vi "Configuration Window.vi"(8 "error in (no error)":errorcluster, 11 "Instrument.Lockin":refnum<class "Instrument.Lockin.lvclass">) -> (0 "error out":errorcluster, 3 "Instrument.Lockin out":refnum<class "Instrument.Lockin.lvclass">)   [LabVIEW 2019, in "Instrument.Lockin.lvlib" / "Instrument.Lockin.lvclass"]
uses:
  Instrument.Lockin.lvclass
  <userlib>/LevyLab/Instrument Framework/Instrument Types/Lockin/Instrument.LockinAPI.lvclass
panel:
  in  "Cancel":bool
  in  "OK":bool
  # "confirm or make changes:"
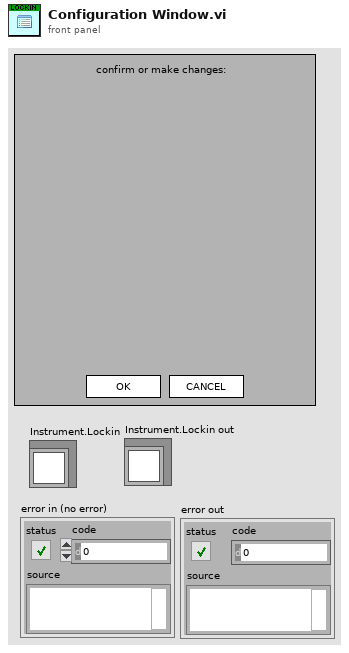
[diagram p1: front panel]
types:
  T1 = enum32{"Invalid", "Standard", "Closed", "Hidden", "Minimized", "Maximized"}
  T2 = enum32{"invalid app kind", "Development System", "Run Time System", "Student Edition", "Embedded LabVIEW", "Evaluation", "Custom"}
  T3 = typedef "Instrument.Lockin.lvlib/Instrument.DAQ.lvclass/Configuration--Cluster.ctl" = cluster{"DAQ":T4, "Channels":T19, "Prefilter":T27, "Offset and Gain":T28, "Amplitude Limit":T31, "DC Limit":T32, "Link Frequencies":T33, "Sweep":T34, "Duty Cycle":T38}
  T4 = typedef "Instrument.Lockin.lvlib/Instrument.DAQ.lvclass/Configuration.DAQ--Cluster.ctl" = cluster{"Sampling":T5, "Simulation mode":T8, "AI":T9, "AO":T14, "Calibration":T16, "Devices":T18[]}
  T5 = typedef "Instrument.Lockin.lvlib/Instrument.DAQ.lvclass/DAQ.Sampling--Cluster.ctl" = cluster{"Sampling":T6, "sample mode":i32, "Fs Mode":T7, "Fs Multiplier":dbl, "Refresh Rate (Hz)":dbl, "Decimation.PreDSP":i32, "Decimation.PostDSP":i32, "Fs.Output":dbl}
  T6 = typedef "Instrument.Lockin.lvlib/Instrument.DAQ.lvclass/DAQ.Sampling.Sampling--Cluster.ctl" = cluster{"Fs":dbl, "#s":i32}
  T7 = typedef "Instrument.Lockin.lvlib/Instrument.DAQ.lvclass/DAQ.Sampling.Fs Mode--enum.ctl" = enum16{"Manual", "Auto Fs", "Max Fs"}
  T8 = typedef "Instrument.Lockin.lvlib/Instrument.DAQ.lvclass/Simulation Mode--enum.ctl" = enum16{"AI = HW simulated", "AI = noise*AO", "AI = waveguide"}
  T9 = typedef "Instrument.Lockin.lvlib/Instrument.DAQ.lvclass/DAQ.Config.AI--Cluster--Array.ctl" = cluster{"Channels":tag, "Coupling":T10, "Range":T11, "terminal configuration":T12, "Type":T13}[]
  T10 = typedef "Instrument.Lockin.lvlib/Instrument.DAQ.lvclass/DAQ.Config.AI.Coupling--enum.ctl" = u16
  T11 = typedef "Instrument.Lockin.lvlib/Instrument.DAQ.lvclass/DAQ.Config.AI.Range--enum.ctl" = enum16{"±0.316", "±1.00", "±3.16", "±10.0", "±31.6", "±42.4", ""}
  T12 = typedef "Instrument.Lockin.lvlib/Instrument.DAQ.lvclass/DAQ.TerminalConfiguration--ring.ctl" = i32
  T13 = typedef "Instrument.Lockin.lvlib/Instrument.DAQ.lvclass/DAQ.Type--enum.ctl" = enum16{"None", "USB-4431", "PXI-446x"}
  T14 = typedef "Instrument.Lockin.lvlib/Instrument.DAQ.lvclass/DAQ.Config.AO--Cluster--Array.ctl" = cluster{"Channels":tag, "Range":T15, "terminal configuration":T12, "Type":T13}[]
  T15 = typedef "Instrument.Lockin.lvlib/Instrument.DAQ.lvclass/DAQ.Config.AO.Range--enum.ctl" = enum16{"±0.1", "±1.0", "±3.5", "±10.0", ""}
  T16 = typedef "Instrument.Lockin.lvlib/Instrument.DAQ.lvclass/DAQ.Calibration--Cluster--Array.ctl" = T17[]
  T17 = typedef "Instrument.Lockin.lvlib/Instrument.DAQ.lvclass/DAQ.Calibration--Cluster.ctl" = cluster{"Active Device":string, "SelfCal.LastDate/Time":dbl, "SelfCal.LastTemp":dbl, "DevTemp":dbl, "calibration due?":bool}
  T18 = typedef "Instrument.Lockin.lvlib/Instrument.DAQ.lvclass/DeviceInfo--Cluster.ctl" = cluster{"DeviceName":string, "DevIsSimulated":bool, "DeviceSerialNumber":string, "ProductType":string, "ProductCategory":i32, "ProductNumber":u32, "ChassisNumber":u32, "SlotNumber":u32, "ChassisName":string, "ChassisSerialNumber":string, "DevTemp":dbl, "SelfCal.LastDate/Time":string, "SelfCal.LastTemp":dbl, "calibration due?":bool}
  T19 = typedef "Instrument.Lockin.lvlib/Instrument.DAQ.lvclass/Configuration.Channels--Cluster.ctl" = cluster{"Cfg_AO":T20, "Cfg_AI":T23, "Cfg_REF":T25}
  T20 = typedef "Instrument.Lockin.lvlib/Instrument.DAQ.lvclass/AO.Channel--Cluster--Array.ctl" = T21[]
  T21 = typedef "Instrument.Lockin.lvlib/Instrument.DAQ.lvclass/AO.Channel--Cluster.ctl" = cluster{"Enable?":bool, "Channel":i32, "Amplitude":dbl, "Offset":dbl, "Frequency":dbl, "Phase":dbl, "Function":T22, "Sweeping?":bool, "Limit AC":bool, "Limit DC?":bool, "Duty Cycle":bool}
  T22 = typedef "Instrument.Lockin.lvlib/Instrument.DAQ.lvclass/AO.Channel.Function--Enum.ctl" = enum16{"sine", "square", "triangle", "saw"}
  T23 = typedef "Instrument.Lockin.lvlib/Instrument.DAQ.lvclass/AI.Channel--Cluster--Array.ctl" = T24[]
  T24 = typedef "Instrument.Lockin.lvlib/Instrument.DAQ.lvclass/AI.Channel--Cluster.ctl" = cluster{"Enable?":bool, "Channel":i32, "References":u16[], "reference index":i32}
  T25 = typedef "Instrument.Lockin.lvlib/Instrument.DAQ.lvclass/REF.Channel--Cluster--Array.ctl" = T26[]
  T26 = typedef "Instrument.Lockin.lvlib/Instrument.DAQ.lvclass/REF.Channel--Cluster.ctl" = cluster{"Enable?":bool, "Channel":i32, "Frequency":dbl, "Phase":dbl, "TC":dbl, "Roll-Off":i32}
  T27 = typedef "Instrument.Lockin.lvlib/Instrument.DAQ.lvclass/Configuration.Prefilter--Cluster.ctl" = cluster{"60 Hz":bool, "Low Pass":bool, "Low Pass Cutoff (Hz)":dbl}
  T28 = typedef "Instrument.Lockin.lvlib/Instrument.DAQ.lvclass/Channel.GainsAndOffsets--Cluster.ctl" = cluster{"Offset_AI":T29, "Gain_AI":T29, "Gain_AO":T29}
  T29 = typedef "Instrument.Lockin.lvlib/Instrument.DAQ.lvclass/Channel.Gain--Cluster--Array.ctl" = T30[]
  T30 = typedef "Instrument.Lockin.lvlib/Instrument.DAQ.lvclass/Channel.Gain--Cluster.ctl" = cluster{"Channel":string, "Gain":dbl}
  T31 = typedef "Instrument.Lockin.lvlib/Instrument.DAQ.lvclass/Configuration.AmplitudeLimit--Cluster.ctl" = cluster{"Limit?":bool, "Limit (V)":dbl}
  T32 = typedef "Instrument.Lockin.lvlib/Instrument.DAQ.lvclass/Configuration.DCLimit--Cluster.ctl" = cluster{"Limit?":bool, "Limit (V)":dbl}
  T33 = typedef "Instrument.Lockin.lvlib/Instrument.DAQ.lvclass/Configuration.LinkFrequencies--Cluster.ctl" = cluster{"Link?":bool, "Frequency (Hz)":dbl}
  T34 = typedef "Instrument.Lockin.lvlib/Instrument.DAQ.lvclass/Sweep.Configuration--Cluster.ctl" = cluster{"Sweep Time (s)":dbl, "Initial Wait (s)":dbl, "Return to Start":bool, "Channels":T35}
  T35 = typedef "Instrument.Lockin.lvlib/Instrument.DAQ.lvclass/Sweep.Channel--Cluster--Array.ctl" = T36[]
  T36 = typedef "Instrument.Lockin.lvlib/Instrument.DAQ.lvclass/Sweep.Channel--Cluster.ctl" = cluster{"Enable?":bool, "Channel":u16, "Start":dbl, "End":dbl, "Pattern":T37, "Table":dbl[]}
  T37 = typedef "Instrument.Lockin.lvlib/Instrument.DAQ.lvclass/Sweep.Pattern--Enum.ctl" = enum16{"Ramp /", "Ramp /\\", "Smooth Ramp _/", "Smooth Ramp _/\\_", "Table"}
  T38 = typedef "Instrument.Lockin.lvlib/Instrument.DAQ.lvclass/Configuration.DutyCycle--Cluster.ctl" = cluster{"Option?":bool, "Duty Cycle (%)":dbl}
  T39 = cluster{"Core":cluster{"Current VI Reference":refnum<vi>, "Close Panel on Exit?":bool}, "Configuration":T3}
  T40 = cluster{"Current VI Reference":refnum<vi>, "Close Panel on Exit?":bool}
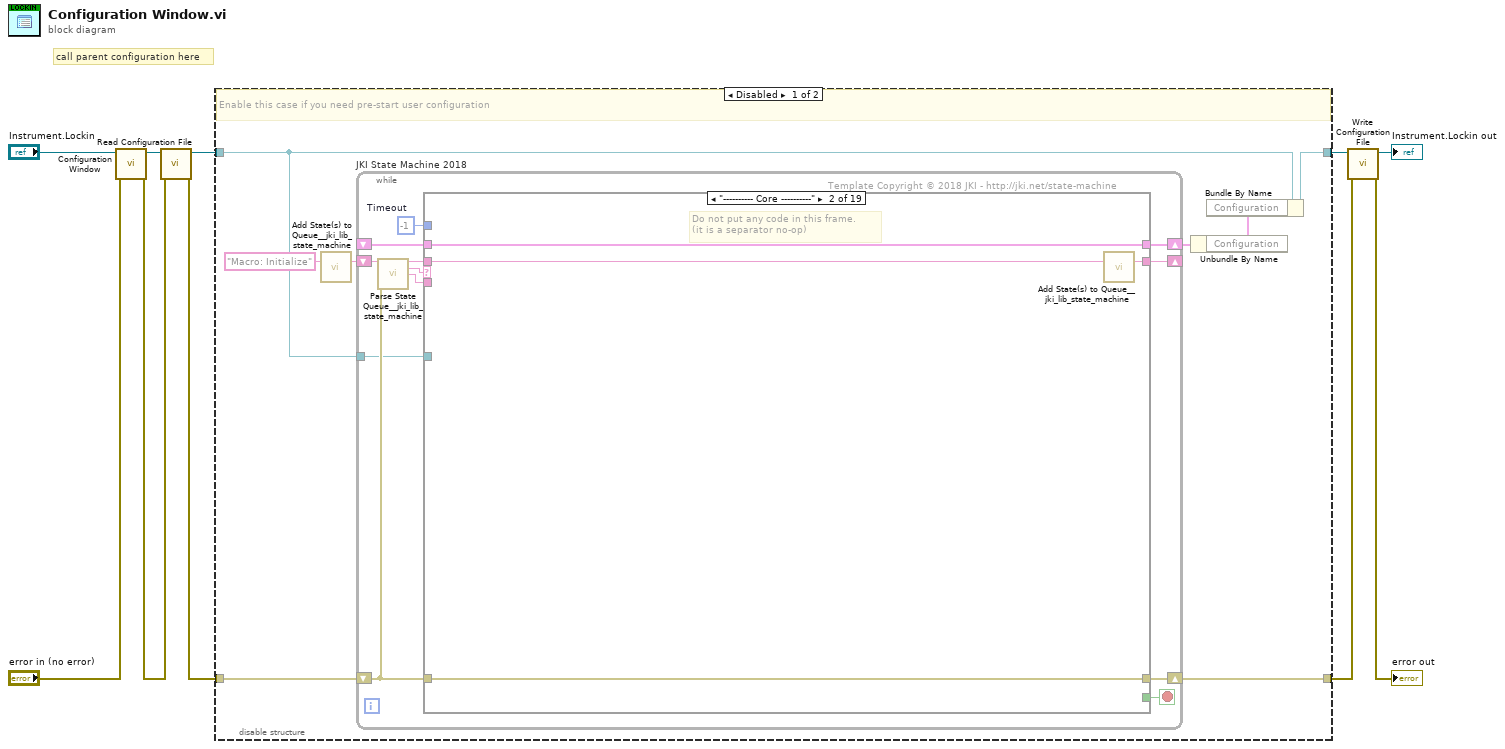
[diagram p0: block diagram]
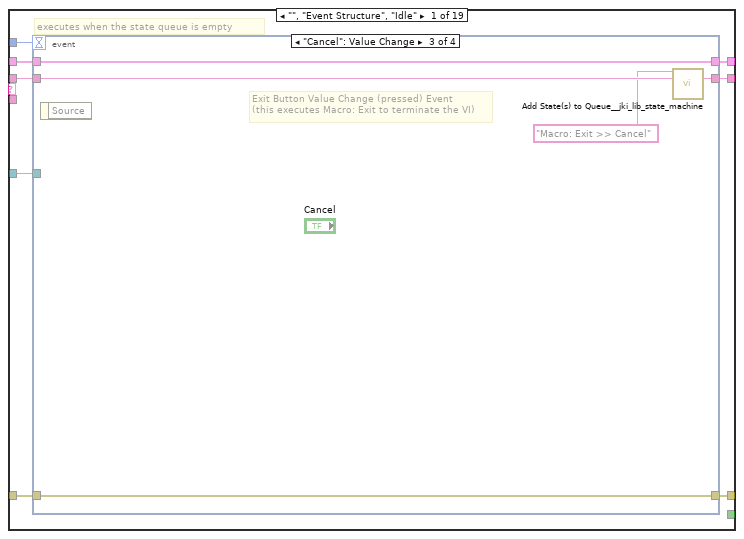
[diagram p2: hidden frame]
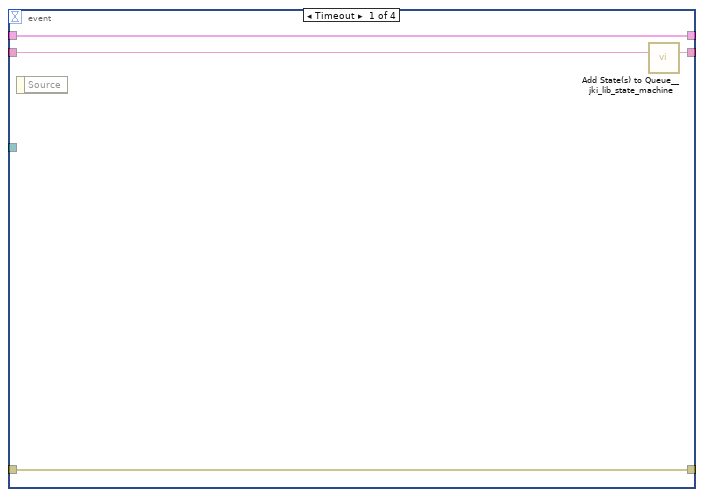
[diagram p3: hidden frame]
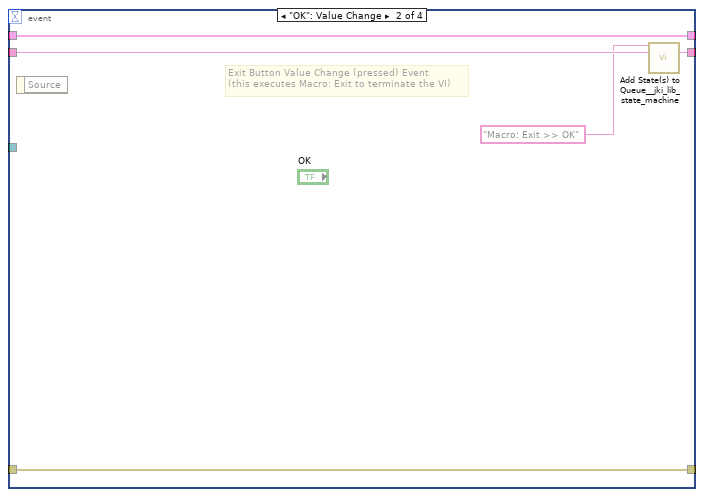
[diagram p4: hidden frame]
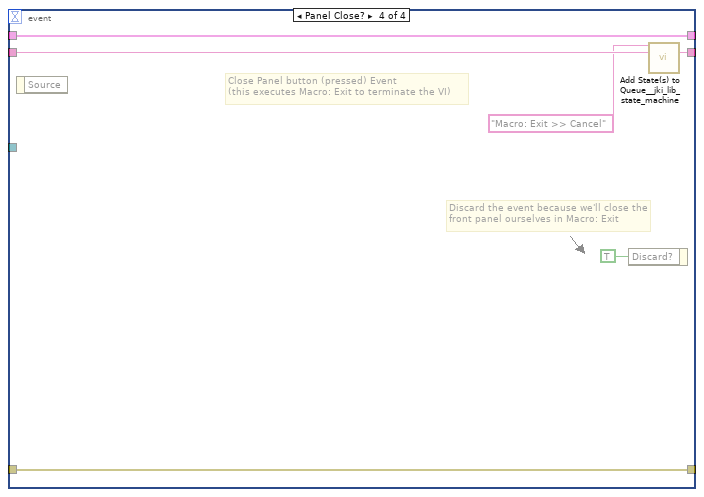
[diagram p5: hidden frame]
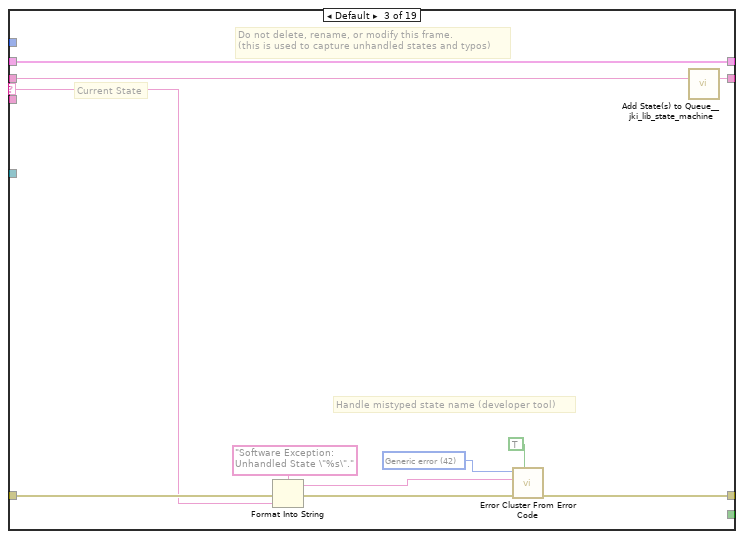
[diagram p6: hidden frame]
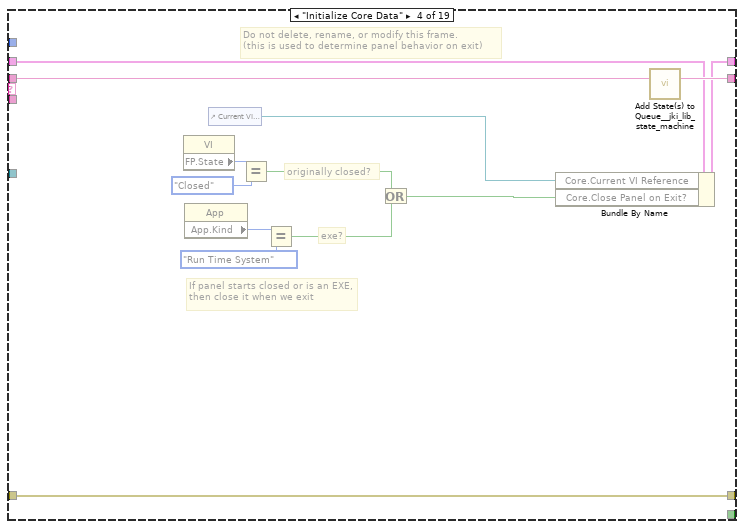
[diagram p7: hidden frame]
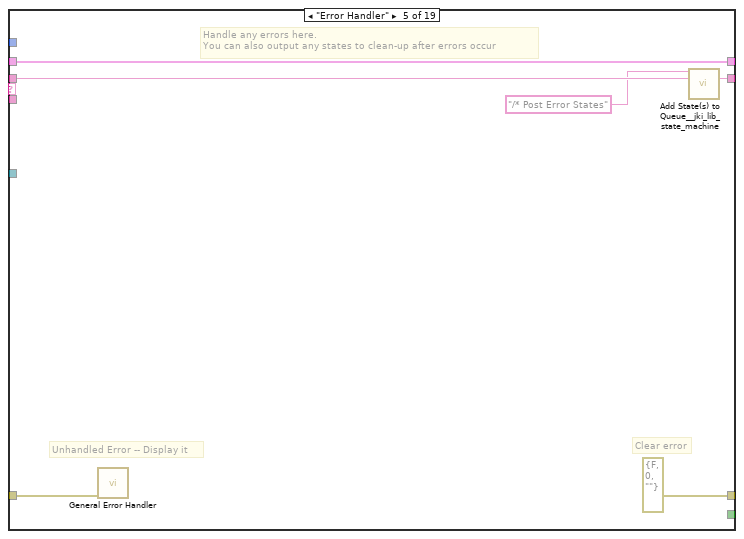
[diagram p8: hidden frame]
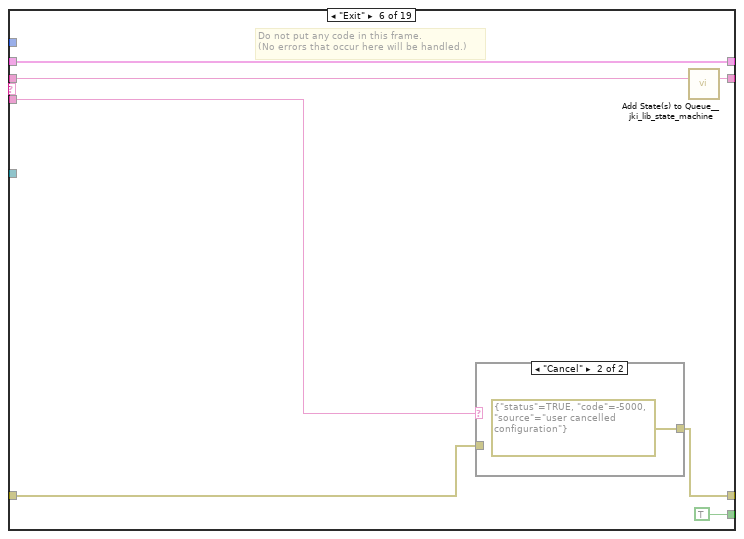
[diagram p9: hidden frame]
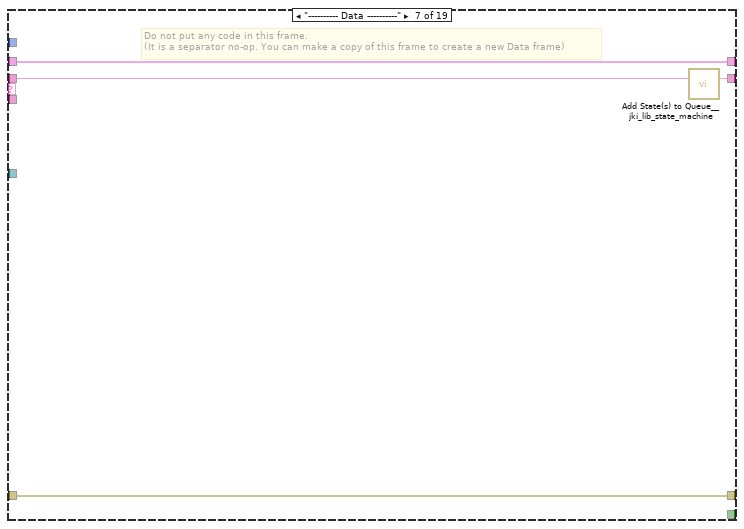
[diagram p11: hidden frame]
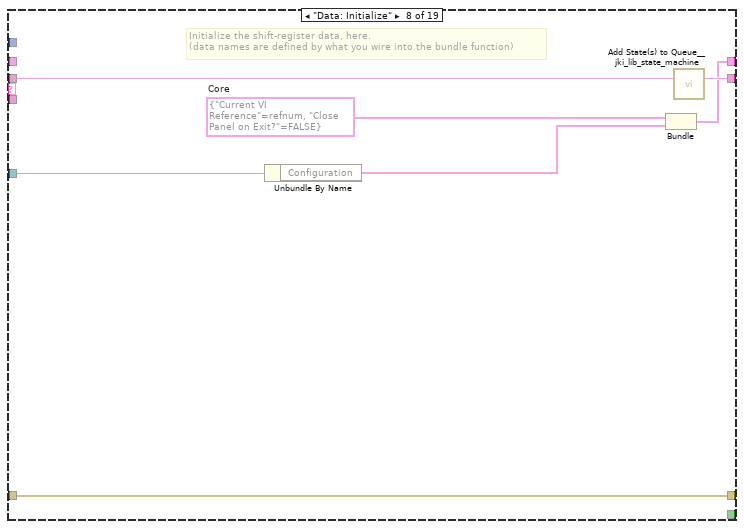
[diagram p12: hidden frame]
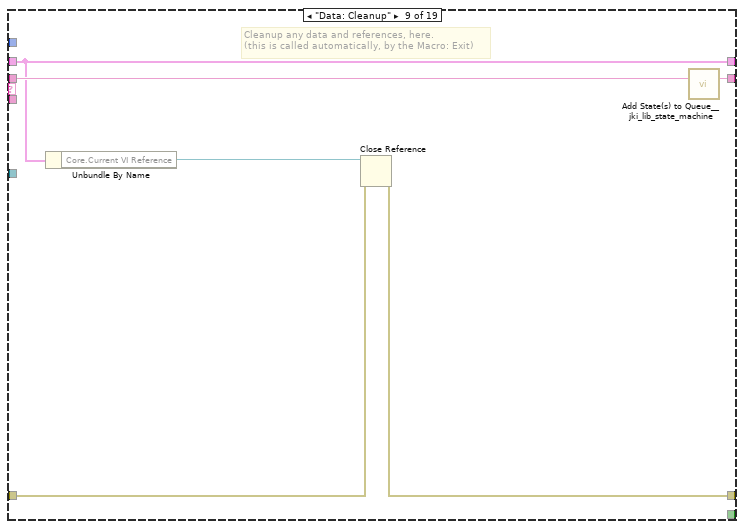
[diagram p13: hidden frame]
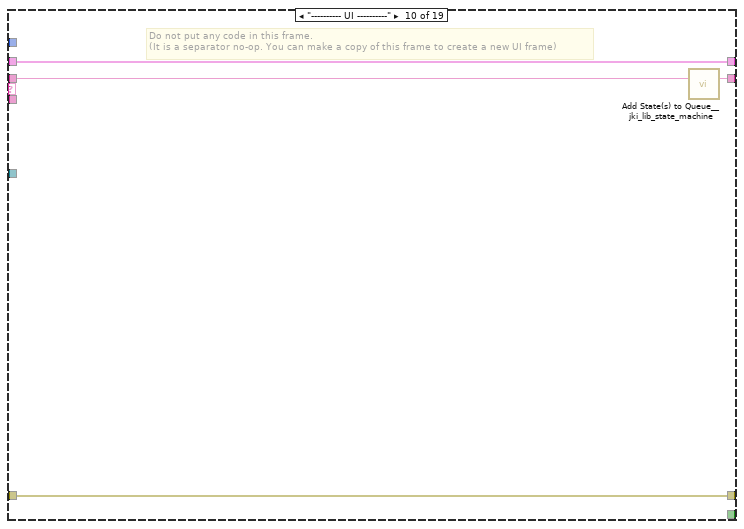
[diagram p14: hidden frame]
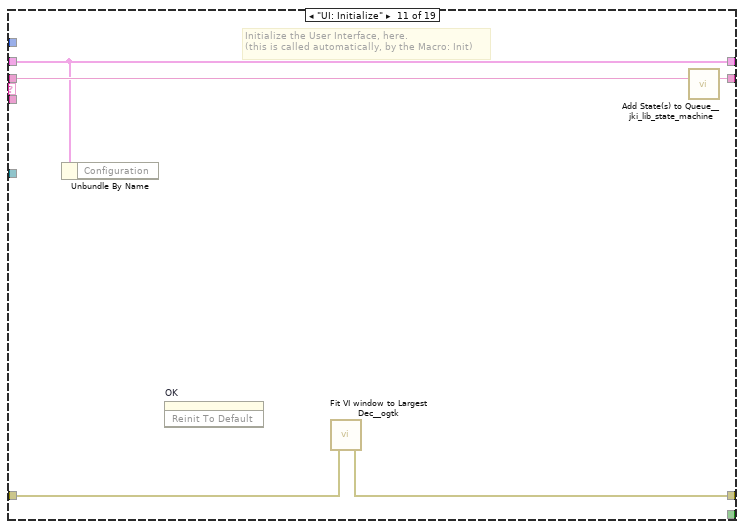
[diagram p15: hidden frame]
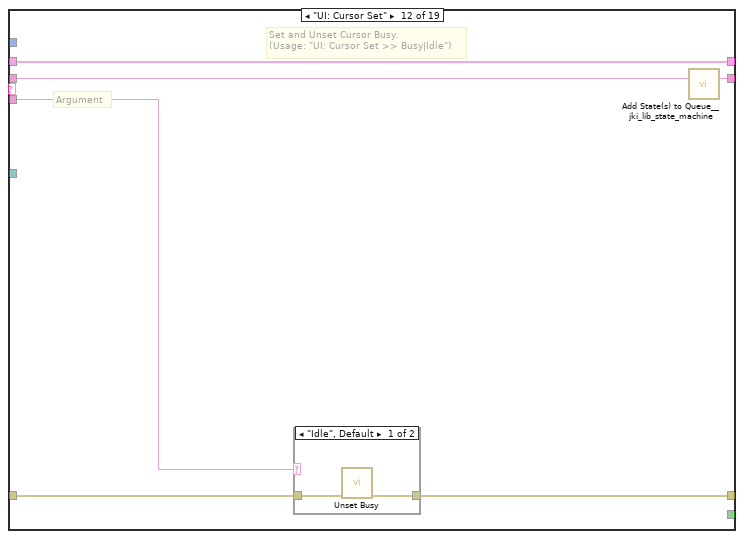
[diagram p16: hidden frame]
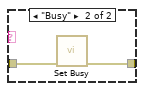
[diagram p17: hidden frame]
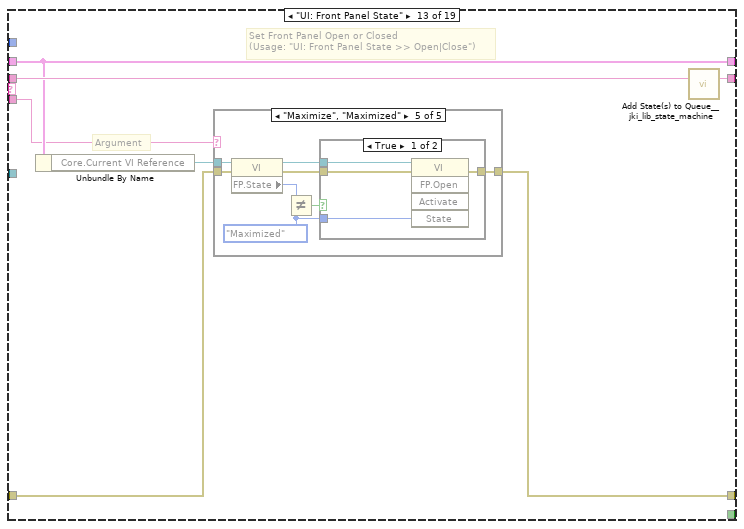
[diagram p18: hidden frame]
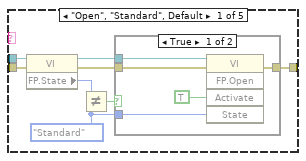
[diagram p19: hidden frame]
diagram:
  # "call parent configuration here"
  n1 = call-parent "Configuration Window.vi"("error in (no error)"="error in (no error)", "Instrument"="Instrument.Lockin") -> ("error out"=w1:errorcluster, "Instrument out"=w3:refnum<class "Instrument.Lockin.lvclass">)  [unwired: 8 in]
  n2 = call-dynamic "Read Configuration File.vi"("error in (no error)"=w1, "Instrument.Lockin"=w3) -> ("error out"=w7:errorcluster, "Instrument.Lockin out"=w6:refnum<class "Instrument.Lockin.lvclass">)  [unwired: 8 in]
  n3 = disable-structure shown="Disabled" {
    disable-tunnel: [w16 w248] -> w8
    disable-tunnel: w7 -> [w15 w248]
    disable-tunnel: w6 -> [w14 w249]
    disable-tunnel: [w13 w249] -> w5
    frame Disabled {
      # "Enable this case if you need pre-start user configuration"
      n4 = call <vilib>:"Add State(s) to Queue__jki_lib_state_machine.vi"("State(s) in (\"\")"="Macro: Initialize") -> ("States Out"=w18:string)  [unwired: 14 in]
      n5 = while "JKI State Machine 2018" {
        shift-right: [w23] -> w12
        shift-left: _ -> [w22]
        shift-right: [w26] -> w16
        shift-left: w15 -> [w20]
        shift-right: [w25] -> _
        shift-left: w18 -> [w27]
        tunnel: w14 -> [w19]
        stop <- w24 stop-if-true
        w21 = -1  # Timeout
        # "Template Copyright © 2018 JKI - http://jki.net/state-machine"
        n6 = call <vilib>:"Parse State Queue__jki_lib_state_machine.vi"("State Queue"=w27, "Error In (no error)"=w20) -> ("Remaining States"=w29:string, "Current State"=w30:string, "Arguments"=w28:string)  [unwired: 11 in]
        n7 = case shown="\"---------- Core ----------\"" w30 {
          selector: w30 -> [_ _ w63 _ _ _ _ _ _ _ _ _ _ _ _ _ _ _ _]
          tunnel: w29 -> [w38 w62 w67 w86 w92 w99 w105 w112 w118 w122 w127 w133 w144 w213 w218 w233 w237 w241 w247]
          tunnel: w28 -> [_ _ _ _ _ w95 _ _ _ _ _ w128 w138 _ _ w222 _ _ _]
          tunnel: w22 -> [w36 w59 w65 w79 w89 w97 w102 _ w113 w119 w123 w131 w140 w210 w215 w230 w234 w238 w243]
          tunnel: [w35 w60 w69 w83 errorcluster {"status"=FALSE, "code"=0, "source"=""} ("error out") w93 w103 w108 w114 w120 w124 w129 w141 w211 w216 w231 w235 w239 w245] -> w26
          tunnel: w20 -> [w34 w60 w68 w83 w88 w94 w103 w108 w115 w120 w125 w130 w142 w211 w216 w231 w235 w239 w245]
          tunnel: [w37 w61 w66 w85 w91 w98 w104 w111 w117 w121 w126 w132 w143 w212 w217 w232 w236 w240 w246] -> w25
          tunnel: [_ _ _ _ _ TRUE _ _ _ _ _ _ _ _ _ _ _ _ _] -> w24
          tunnel: [w33 w59 w65 w84 w89 w97 w102 w110 w113 w119 w123 w131 w140 w210 w215 w230 w234 w238 w244] -> w23
          tunnel: w21 -> [w32 _ _ _ _ _ _ _ _ _ _ _ _ _ _ _ _ _ _]
          tunnel: w19 -> [w31 _ _ _ _ _ _ w107 _ _ _ _ _ _ _ _ _ _ _]
          frame "", "Event Structure", "Idle" {
            # "executes when the state queue is empty"
            n8 = event shown="[2] \"Cancel\": Value Change" {
              selector: _ -> [_ _ _ _]
              dyn-events: _ -> [_ _ _ _]
              timeout: w32 -> [_ _ _ _]
              tunnel: w38 -> [w42 w47 w52 w58]
              tunnel: [w41 w46 w51 w57] -> w37
              tunnel: w36 -> [w39 w44 w49 w55]
              tunnel: [w40 w45 w50 w56] -> w35
              tunnel: w34 -> [w40 w45 w50 w56]
              tunnel: [w39 w44 w49 w55] -> w33
              tunnel: w31 -> [_ _ _ _]
              event Timeout {
                n9 = event-data() -> ()  [unwired: 1 in, 1 out]
                n10 = call <vilib>:"Add State(s) to Queue__jki_lib_state_machine.vi"("State(s) in (\"\")"=w42) -> ("States Out"=w41:string)  [unwired: 14 in]
              }
              event "OK": Value Change {
                # "Exit Button Value Change (pressed) Event\n(this executes Macro: Exit to terminate the VI)"
                n11 = event-data() -> ()  [unwired: 1 in, 1 out]
                n12 = call <vilib>:"Add State(s) to Queue__jki_lib_state_machine.vi"("State(s) in Front (\"\")"="Macro: Exit >> OK", "State(s) in (\"\")"=w47) -> ("States Out"=w46:string)  [unwired: 13 in]
              }
              event "Cancel": Value Change {
                # "Exit Button Value Change (pressed) Event\n(this executes Macro: Exit to terminate the VI)"
                n13 = event-data() -> ()  [unwired: 1 in, 1 out]
                n14 = call <vilib>:"Add State(s) to Queue__jki_lib_state_machine.vi"("State(s) in Front (\"\")"="Macro: Exit >> Cancel", "State(s) in (\"\")"=w52) -> ("States Out"=w51:string)  [unwired: 13 in]
              }
              event Panel Close? {
                # "Discard the event because we'll close the front panel ourselves in Macro: Exit"
                # "Close Panel button (pressed) Event\n(this executes Macro: Exit to terminate the VI)"
                n15 = event-data() -> ()  [unwired: 1 in, 1 out]
                n16 = event-data("Discard?"=TRUE) -> ()  [unwired: 1 in, 1 out]
                n17 = call <vilib>:"Add State(s) to Queue__jki_lib_state_machine.vi"("State(s) in Front (\"\")"="Macro: Exit >> Cancel", "State(s) in (\"\")"=w58) -> ("States Out"=w57:string)  [unwired: 13 in]
              }
            }
          }
          frame "---------- Core ----------" {
            # "Do not put any code in this frame.\n(it is a separator no-op)"
            n18 = call <vilib>:"Add State(s) to Queue__jki_lib_state_machine.vi"("State(s) in (\"\")"=w62) -> ("States Out"=w61:string)  [unwired: 14 in]
          }
          frame Default {
            w72 = 42 items=["No error", "Argument error", "Memory is full", "Out of zone", "End of file", "File already open", "Generic file I/O error", "File not found", "File permission error", "Disk is full", "Duplicate path", "Too many files open", "System feature not enabled", "Resource file not found", "Cannot add resource", "Resource not found", "Image not found", "Image memory error", "Pen does not exist", "Config type invalid", "Config token not found", "Config parse error", "Config memory error", "Bad external code format", "Bad external code offset", "External code not present", "Null window", "Destroy window error", "Null menu", "Print aborted", "Bad print record", "Print driver error", "Windows error during printing", "Memory error during printing", "Print dialog error", "Generic print error", "Invalid device refnum", "Device not found", "Device parameter error", "Device unit error", "Cannot open device", "Device call aborted", "Generic error", "Cancelled by user", "Object ID too low", "Object ID too high", "Object not in heap", "Unknown heap", "Unknown object (invalid DefProc)", "Unknown object (DefProc not in table)", "Message out of range", "Invalid (null) method", "Unknown message", "Manager call not supported", "Bad address", "Network operation in progress", "Network operation timed out", "Connection is busy", "Network attribute not supported", "Network error", "Address in use", "System out of memory", "Connection aborted", "Connection refused", "Not connected", "Already connected", "Connection closed", "Initialization error (interapplication manager)", "Bad occurrence", "Wait on unbound occurrence handler", "Occurrence queue overflow", "Datalog type conflict", "Unused", "Unrecognized type (interapplication manager)", "Memory corrupt", "Failed to make temporary DLL", "Old CIN version", "Drag socket not found", "Failed to load drop-object", "Failed to register OLE object", "Failed to release OLE object", "Format specifier type mismatch", "Unknown format specifier", "Too few format specifiers", "Too many format specifiers", "Scan failed", "Newer CIN version", "Error converting to variant", "Runtime menu error", "Password tampered", "Variant attribute not found", "Incompatible variant data type", "Event data is not available", "Event Store is not present", "Occurrence is not found", "Event Queue is not created", "Event info is not available", "Refnum passed is NULL", "Error retrieving Class GUID", "Error retrieving CoClass GUID", "Error retrieving TypeLib GUID.", "Bad built application magic bytes.", "Specific driver is different from the specific driver associated with the Logical Name.", "There is no session opened to the class driver.", "Max Error", "MAX - Error with config objects", "MAX - Error loading configuration", "MAX - Group not supported"]
            # "Current State"
            # "Do not delete, rename, or modify this frame.\n(this is used to capture unhandled states and typos)"
            # "Handle mistyped state name (developer tool)"
            n19 = Format Into String(format string="Software Exception: Unhandled State \"%s\"." ("message"), error in=w68, w63) -> (resulting string=w71:string, error out=w70:errorcluster)  [unwired: 1 in]
            n20 = call <vilib>:"Error Cluster From Error Code.vi"("show call chain? (False)"=TRUE, "error in (no error)"=w70, "error message (\"\")"=w71, "error code (0)"=w72) -> ("error out"=w69:errorcluster)  [unwired: 5 in]
            n21 = call <vilib>:"Add State(s) to Queue__jki_lib_state_machine.vi"("State(s) in (\"\")"=w67) -> ("States Out"=w66:string)  [unwired: 14 in]
          }
          frame "Initialize Core Data" {
            # "Do not delete, rename, or modify this frame.\n(this is used to determine panel behavior on exit)"
            # "originally closed?"
            # "exe?"
            # "If panel starts closed or is an EXE, then close it when we exit"
            n22 = property class="VI"() -> ("FP.State"=w76:T1)  [unwired: 2 in, 2 out]
            n23 = property class="App"() -> ("App.Kind"=w82:T2)  [unwired: 2 in, 2 out]
            n24 = control-ref of="Current VI Reference"() -> (w77:refnum<vi>)
            n25 = Equal?(x=w76, y=T1."Closed" ("Front Panel Window:State")) -> (x = y?=w74:bool)
            n26 = Equal?(x=w82, y=T2."Run Time System" ("Application:Kind")) -> (x = y?=w80:bool)
            n27 = Or(x=w74, y=w80) -> (x .or. y?=w78:bool)
            n28 = Bundle By Name(cluster=w79, "Core.Current VI Reference"=w77, "Core.Close Panel on Exit?"=w78) -> (w84:T39)
            n29 = call <vilib>:"Add State(s) to Queue__jki_lib_state_machine.vi"("State(s) in (\"\")"=w86) -> ("States Out"=w85:string)  [unwired: 14 in]
          }
          frame "Error Handler" {
            # "Unhandled Error -- Display it"
            # "Handle any errors here.\nYou can also output any states to clean-up after errors occur"
            # "Clear error"
            n30 = call <vilib>:"General Error Handler.vi"("error in (no error)"=w88) -> ()  [unwired: 10 in, 5 out]
            n31 = call <vilib>:"Add State(s) to Queue__jki_lib_state_machine.vi"("State(s) in Front (\"\")"="/* Post Error States", "State(s) in (\"\")"=w92) -> ("States Out"=w91:string)  [unwired: 13 in]
          }
          frame "Exit" {
            # "Do not put any code in this frame.\n(No errors that occur here will be handled.)"
            n32 = case shown="\"Cancel\"" w95 {
              tunnel: w94 -> [w100 _]
              tunnel: [w100 errorcluster {"status"=TRUE, "code"=-5000, "source"="user cancelled configuration"} ("error in (no error)")] -> w93
              frame "OK", Default {
              }
              frame "Cancel" {
              }
            }
            n33 = call <vilib>:"Add State(s) to Queue__jki_lib_state_machine.vi"("State(s) in (\"\")"=w99) -> ("States Out"=w98:string)  [unwired: 14 in]
          }
          frame "---------- Data ----------" {
            # "Do not put any code in this frame.\n(It is a separator no-op. You can make a copy of this frame to create a new Data frame)"
            n34 = call <vilib>:"Add State(s) to Queue__jki_lib_state_machine.vi"("State(s) in (\"\")"=w105) -> ("States Out"=w104:string)  [unwired: 14 in]
          }
          frame "Data: Initialize" {
            w109 = T40 {"Current VI Reference"=refnum, "Close Panel on Exit?"=FALSE}  # Core
            # "Initialize the shift-register data, here.\n(data names are defined by what you wire into the bundle function)"
            n35 = Unbundle By Name(w107) -> ("Configuration"=w106:T3)
            n36 = Bundle("Core"=w109, "Configuration"=w106) -> (w110:T39)  [unwired: 1 in]
            n37 = call <vilib>:"Add State(s) to Queue__jki_lib_state_machine.vi"("State(s) in (\"\")"=w112) -> ("States Out"=w111:string)  [unwired: 14 in]
          }
          frame "Data: Cleanup" {
            # "Cleanup any data and references, here.\n(this is called automatically, by the Macro: Exit)"
            n38 = Unbundle By Name(w113) -> ("Core.Current VI Reference"=w116:refnum<vi>)
            n39 = Close Reference(reference=w116, error in (no error)=w115) -> (error out=w114:errorcluster)
            n40 = call <vilib>:"Add State(s) to Queue__jki_lib_state_machine.vi"("State(s) in (\"\")"=w118) -> ("States Out"=w117:string)  [unwired: 14 in]
          }
          frame "---------- UI ----------" {
            # "Do not put any code in this frame.\n(It is a separator no-op. You can make a copy of this frame to create a new UI frame)"
            n41 = call <vilib>:"Add State(s) to Queue__jki_lib_state_machine.vi"("State(s) in (\"\")"=w122) -> ("States Out"=w121:string)  [unwired: 14 in]
          }
          frame "UI: Initialize" {
            # "Initialize the User Interface, here.\n(this is called automatically, by the Macro: Init)"
            n42 = Unbundle By Name(w123) -> ()  [unwired: 1 out]
            n43 = invoke on="OK" class="Bool" method="Reinit To Default"() -> ()  [unwired: 3 in, 3 out]
            n44 = call <userlib>:"Fit VI window to Largest Dec__ogtk.vi"("error in (no error)"=w125) -> ("error out"=w124:errorcluster)  [unwired: 5 in, 1 out]
            n45 = call <vilib>:"Add State(s) to Queue__jki_lib_state_machine.vi"("State(s) in (\"\")"=w127) -> ("States Out"=w126:string)  [unwired: 14 in]
          }
          frame "UI: Cursor Set" {
            # "Argument"
            # "Set and Unset Cursor Busy.\n(Usage: \"UI: Cursor Set >> Busy|Idle\")"
            n46 = case shown="\"Idle\", Default" w128 {
              tunnel: w130 -> [w135 w137]
              tunnel: [w134 w136] -> w129
              frame "Idle", Default {
                n47 = call <vilib>:"Unset Busy.vi"("error in (no error)"=w135) -> ("error out"=w134:errorcluster)  [unwired: 10 in]
              }
              frame "Busy" {
                n48 = call <vilib>:"Set Busy.vi"("error in (no error)"=w137) -> ("error out"=w136:errorcluster)  [unwired: 9 in, 1 out]
              }
            }
            n49 = call <vilib>:"Add State(s) to Queue__jki_lib_state_machine.vi"("State(s) in (\"\")"=w133) -> ("States Out"=w132:string)  [unwired: 14 in]
          }
          frame "UI: Front Panel State" {
            # "Argument"
            # "Set Front Panel Open or Closed\n(Usage: \"UI: Front Panel State >> Open|Close\")"
            n50 = Unbundle By Name(w140) -> ("Core.Current VI Reference"=w139:refnum<vi>)
            n51 = case shown="\"Maximize\", \"Maximized\"" w138 {
              tunnel: w142 -> [w150 w165 w176 w189 w202]
              tunnel: [w152 w166 w178 w191 w204] -> w141
              tunnel: w139 -> [w151 w163 w177 w190 w203]
              frame "Open", "Standard", Default {
                w145 = T1."Standard" ("State")
                n52 = property class="VI"(reference=w151, error in=w150) -> (reference out=w148:refnum<vi>, error out=w149:errorcluster, "FP.State"=w147:T1)
                n53 = Not Equal?(x=w147, y=w145) -> (x != y?=w146:bool)
                n54 = case shown="True" w146 {
                  tunnel: [w156 w158] -> w152
                  tunnel: w149 -> [w155 w158]
                  tunnel: w148 -> [w154 _]
                  tunnel: w145 -> [w153 _]
                  frame True {
                    n55 = invoke class="VI" method="FP.Open"(reference=w154, error in=w155, "Activate"=TRUE, "State"=w153) -> (error out=w156:errorcluster)  [unwired: 1 in, 4 out]
                  }
                  frame False {
                  }
                }
              }
              frame "Close", "Closed" {
                n56 = property class="VI"(reference=w163, error in=w165) -> (reference out=w162:refnum<vi>, error out=w164:errorcluster, "FP.State"=w160:T1)
                n57 = Not Equal?(x=w160, y=T1."Closed" ("Front Panel Window:State")) -> (x != y?=w159:bool)
                n58 = case shown="True" w159 {
                  tunnel: [w167 w170] -> w166
                  tunnel: w164 -> [w167 w169]
                  tunnel: w162 -> [_ w168]
                  frame False {
                  }
                  frame True {
                    n59 = invoke class="VI" method="FP.Close"(reference=w168, error in=w169) -> (error out=w170:errorcluster)  [unwired: 1 in, 2 out]
                  }
                }
              }
              frame "Hidden", "Hide" {
                w171 = T1."Hidden" ("State")
                n60 = property class="VI"(reference=w177, error in=w176) -> (reference out=w174:refnum<vi>, error out=w175:errorcluster, "FP.State"=w173:T1)
                n61 = Not Equal?(x=w173, y=w171) -> (x != y?=w172:bool)
                n62 = case shown="True" w172 {
                  tunnel: [w182 w183] -> w178
                  tunnel: w175 -> [w181 w183]
                  tunnel: w174 -> [w180 _]
                  tunnel: w171 -> [w179 _]
                  frame True {
                    n63 = invoke class="VI" method="FP.Open"(reference=w180, error in=w181, "State"=w179) -> (error out=w182:errorcluster)  [unwired: 2 in, 4 out]
                  }
                  frame False {
                  }
                }
              }
              frame "Minimize", "Minimized" {
                w184 = T1."Minimized" ("State")
                n64 = property class="VI"(reference=w190, error in=w189) -> (reference out=w187:refnum<vi>, error out=w188:errorcluster, "FP.State"=w186:T1)
                n65 = Not Equal?(x=w186, y=w184) -> (x != y?=w185:bool)
                n66 = case shown="True" w185 {
                  tunnel: [w195 w196] -> w191
                  tunnel: w188 -> [w194 w196]
                  tunnel: w187 -> [w193 _]
                  tunnel: w184 -> [w192 _]
                  frame True {
                    n67 = invoke class="VI" method="FP.Open"(reference=w193, error in=w194, "State"=w192) -> (error out=w195:errorcluster)  [unwired: 2 in, 4 out]
                  }
                  frame False {
                  }
                }
              }
              frame "Maximize", "Maximized" {
                w197 = T1."Maximized" ("State")
                n68 = property class="VI"(reference=w203, error in=w202) -> (reference out=w200:refnum<vi>, error out=w201:errorcluster, "FP.State"=w199:T1)
                n69 = Not Equal?(x=w199, y=w197) -> (x != y?=w198:bool)
                n70 = case shown="True" w198 {
                  tunnel: [w208 w209] -> w204
                  tunnel: w201 -> [w207 w209]
                  tunnel: w200 -> [w206 _]
                  tunnel: w197 -> [w205 _]
                  frame True {
                    n71 = invoke class="VI" method="FP.Open"(reference=w206, error in=w207, "State"=w205) -> (error out=w208:errorcluster)  [unwired: 2 in, 4 out]
                  }
                  frame False {
                  }
                }
              }
            }
            n72 = call <vilib>:"Add State(s) to Queue__jki_lib_state_machine.vi"("State(s) in (\"\")"=w144) -> ("States Out"=w143:string)  [unwired: 14 in]
          }
          frame "---------- Macro ----------" {
            # "Do not put any code in this frame.\n(It is a separator no-op. You can make a copy of this frame to create a new Macro frame)"
            n73 = call <vilib>:"Add State(s) to Queue__jki_lib_state_machine.vi"("State(s) in (\"\")"=w213) -> ("States Out"=w212:string)  [unwired: 14 in]
          }
          frame "Macro: Initialize" {
            w214 = "Data: Initialize\nInitialize Core Data\nUI: Initialize\nUI: Front Panel State >> Open\nConfiguration: Read"  # Data: Initialize Initialize Core Data UI: Initialize UI: Front Panel State >> Open Configuration: Read
            # "Initialization Macro\n(This is called once, when the VI starts)"
            n74 = call <vilib>:"Add State(s) to Queue__jki_lib_state_machine.vi"("State(s) in Front (\"\")"=w214, "State(s) in (\"\")"=w218) -> ("States Out"=w217:string)  [unwired: 13 in]
          }
          frame "Macro: Exit" {
            # "Exit Macro\n(This is called once, when the VI exits)"
            n75 = Unbundle By Name(w230) -> ("Core.Close Panel on Exit?"=w229:bool)
            n76 = call <vilib>:"Build State String with Arguments__JKI_lib_State_Machine.vi"("Arguments (\"\")"=w222, "State"="Exit") -> ("State with Arguments"=w220:string)  [unwired: 4 in]
            n77 = Select(t="UI: Front Panel State >> Close", s=w229, f="") -> (s? t:f=w226:string)
            n78 = call <vilib>:"Add State(s) to Queue__jki_lib_state_machine.vi"("State(s) in Front (\"\")"="Data: Cleanup", "State(s) at Back (\"\")"=w220) -> ("States Out"=w219:string)  [unwired: 13 in]
            n79 = call <vilib>:"Add State(s) to Queue__jki_lib_state_machine.vi"("State(s) in Front (\"\")"="Configuration: Write", "State(s) in (\"\")"=w226, "State(s) at Back (\"\")"=w219) -> ("States Out"=w225:string)  [unwired: 12 in]
            n80 = call <vilib>:"Add State(s) to Queue__jki_lib_state_machine.vi"("State(s) in Front (\"\")"=w225, "State(s) in (\"\")"=w233) -> ("States Out"=w232:string)  [unwired: 13 in]
          }
          frame "---------- Configuration ----------" {
            # "Template Separator\n(You can make a copy of, or modify, this frame)"
            n81 = call <vilib>:"Add State(s) to Queue__jki_lib_state_machine.vi"("State(s) in (\"\")"=w237) -> ("States Out"=w236:string)  [unwired: 14 in]
          }
          frame "Configuration: Read" {
            # "Your code here.\n(You can make a copy of, or modify, this frame)"
            n82 = Unbundle By Name(w238) -> ()  [unwired: 1 out]
            n83 = call <vilib>:"Add State(s) to Queue__jki_lib_state_machine.vi"("State(s) in (\"\")"=w241) -> ("States Out"=w240:string)  [unwired: 14 in]
          }
          frame "Configuration: Write" {
            n84 = Unbundle By Name(w243) -> ("Configuration"=w242:T3)
            n85 = Bundle By Name(cluster=w243, "Configuration"=w242) -> (w244:T39)
            n86 = call <vilib>:"Add State(s) to Queue__jki_lib_state_machine.vi"("State(s) in (\"\")"=w247) -> ("States Out"=w246:string)  [unwired: 14 in]
          }
        }
      }
      n87 = Unbundle By Name(w12) -> ("Configuration"=w11:T3)
      n88 = Bundle By Name(cluster=w14, "Configuration"=w11) -> (w13:refnum<class "Instrument.Lockin.lvclass">)
    }
    frame Enabled {
    }
  }
  n89 = call-dynamic "Write Configuration File.vi"("error in (no error)"=w8, "Instrument.Lockin"=w5) -> ("error out"=→"error out":errorcluster, "Instrument.Lockin out"=→"Instrument.Lockin out":refnum<class "Instrument.Lockin.lvclass">)  [unwired: 8 in]
